vi "Display PDF File in Dialog Box LV 2012 NI Verified.vi"(8 "error in (no error)":errorcluster, 11 "PDF file":path) -> (0 "error out":errorcluster)   [LabVIEW 2020]
doc: "Use this VI to display a PDF document in a dialog box.\nIn the <B>PDF file</B> text box, enter the path to the PDF you want to display, or click the <B>Browse</B> button to navigate to a file.\nClick the <B>Run</B> button to view the PDF in the <B>PDF display</B>.\nClick the <B>Stop</B> button to stop the VI and remove the PDF from display."
panel:
  in  "STOP":bool
  in  "AcroPDF":refnum<k7>(container)
  # "Overview: This example demonstrates how to open a PDF file and view it within a dialog box on the LabVIEW front panel \nRequirements: LabVIEW 2012 (or compatible)\nInstructions: \n1. Set PDF file path control properly, by browsing to an existing PDF file \n2. Run the VI\n3. Stop the VI by pressing STOP button"
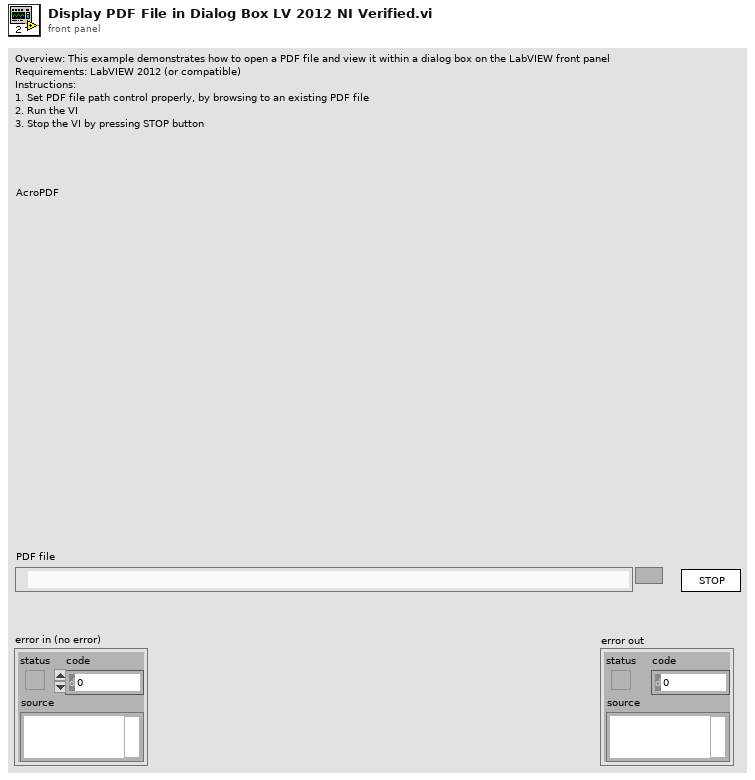
[diagram p1: front panel]
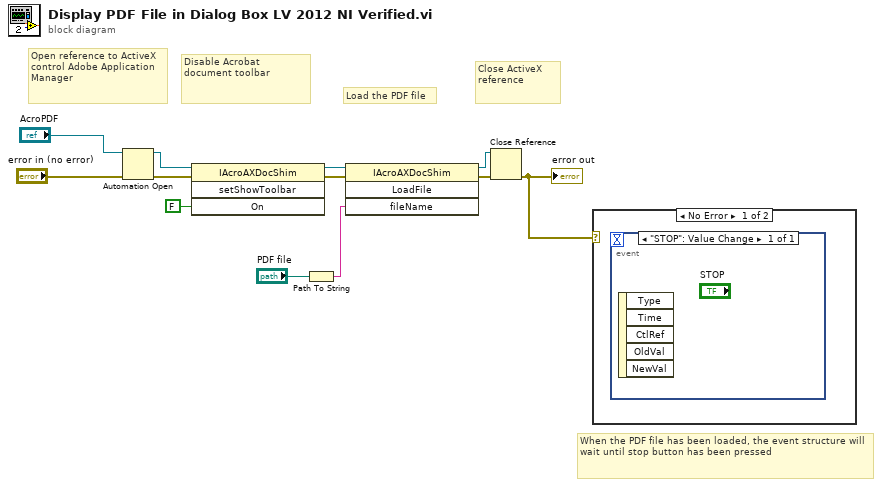
[diagram p0: block diagram]
diagram:
  # "Disable Acrobat document toolbar"
  # "Load the PDF file"
  # "Close ActiveX reference"
  # "Open reference to ActiveX control Adobe Application Manager"
  # "When the PDF file has been loaded, the event structure will wait until stop button has been pressed"
  n1 = Automation Open(error in (no error)="error in (no error)", Automation Refnum="AcroPDF") -> (Automation Refnum=w3:refnum<k7>, error out=w1:errorcluster)  [unwired: 2 in]
  n2 = invoke class="IAcroAXDocShim" method="setShowToolbar"(reference=w3, error in=w1, "On"=FALSE) -> (reference out=w6:refnum<k7>, error out=w5:errorcluster)  [unwired: 1 in, 2 out]
  n3 = Path To String(path="PDF file") -> (string=w10:string)
  n4 = invoke class="IAcroAXDocShim" method="LoadFile"(reference=w6, error in=w5, "fileName"=w10) -> (reference out=w12:refnum<k7>, error out=w11:errorcluster)  [unwired: 1 in, 2 out]
  n5 = Close Reference(reference=w12, error in (no error)=w11) -> (error out=w8:errorcluster)
  "error out" <- w8
  n6 = case shown="No Error" w8 {
    frame No Error {
      n7 = event shown="[0] \"STOP\": Value Change" {
        selector: _ -> [_]
        dyn-events: _ -> [_]
        timeout: _ -> [_]
        event "STOP": Value Change {
          n8 = event-data() -> ()  [unwired: 1 in, 5 out]
        }
      }
    }
    frame Error {
    }
  }
